vi "Send Configure Data Marker [DM].vi"(5 "Destination Terminal (None)":string(combo) caption="destination terminal (None)", 6 "Source Channel (\"\")":string="CHANNEL1" caption="source channel (\"CHANNEL1\")", 7 "Message Priority (Normal)":T1=enum."Normal", 8 "error in (no error)":errorcluster, 9 "Marker Name (\"\")":string caption="marker name (\"\")", 10 "Bit Position":i32 caption="bit position" format="%.0g", 11 "Message Enqueuer":refnum<class "Message Enqueuer.lvclass">) -> (0 "error out":errorcluster, 3 "Message Enqueuer out":refnum<class "Message Enqueuer.lvclass">)   [LabVIEW 2013, in "CS++Fgen.lvlib" / "Configure Data Marker [DM] Msg.lvclass"]
doc: "This VI sends the message to an actor."
uses:
  Configure Data Marker [DM] Msg.lvclass
  <vilib>/ActorFramework/Message Enqueuer/Message Enqueuer.lvclass
  <vilib>/ActorFramework/Message Enqueuer/Message Priority.ctl
  Configure Data Marker [DM] Msg.lvclass/Configure Data Marker [DM] Msg.ctl
  <vilib>/ActorFramework/Message Enqueuer/Message Enqueuer.lvclass/Message Enqueuer.ctl
  <vilib>/ActorFramework/Message Priority Queue/Priority Enqueue.vi
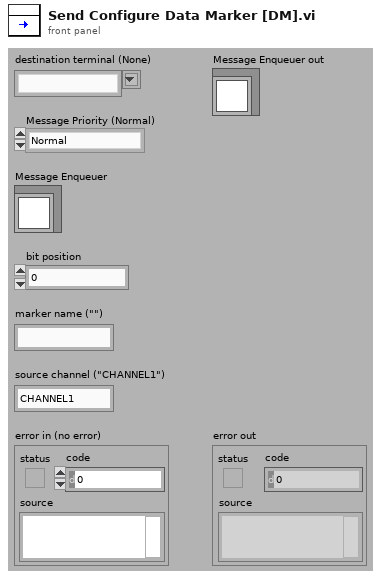
[diagram p1: front panel]
types:
  T1 = typedef "Actor Framework.lvlib/Message Enqueuer.lvclass/Message Priority.ctl" = enum16{"Low", "Normal", "High"}
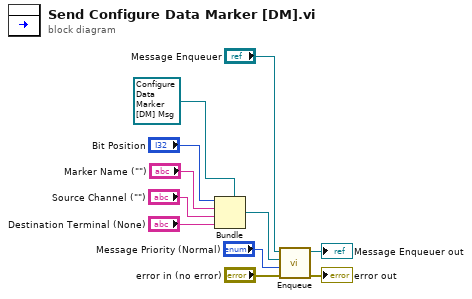
[diagram p0: block diagram]
diagram:
  n1 = Bundle(cluster=refnum<class "Configure Data Marker [DM] Msg.lvclass"> refnum ("Object"), "Bit Position", "Marker Name (\"\")", "Source Channel (\"\")", "Destination Terminal (None)") -> (w7:refnum<class "Configure Data Marker [DM] Msg.lvclass">)
  n2 = call <vilib>:"Enqueue.vi"("error in (no error)"="error in (no error)", "Message Priority (Normal)"="Message Priority (Normal)", "Message"=w7, "Message Enqueuer in"="Message Enqueuer") -> ("error out"=→"error out":errorcluster, "Message Enqueuer out"=→"Message Enqueuer out":refnum<class "Message Enqueuer.lvclass">)  [unwired: 6 in]
